vi "svl_Running Equivalent Continuous Sound Level (1 Ch).vi"(6 "integration time [s]":dbl=1.0 format="%.2f", 8 "error in (no error)":errorcluster, 9 "processing state":T1(ring)=enum."Restart averaging", 11 "scaled signal":waveform(dbl)={"t0"=timestamp(0 s since 1904-01-01), "dt"=0.0, "Y"=[]}) -> (0 "error out":errorcluster, 3 "Running Leq":dbl format="%.2f", 4 "actual integration time [s]":dbl=1.0 format="%.2f")   [LabVIEW 2017]
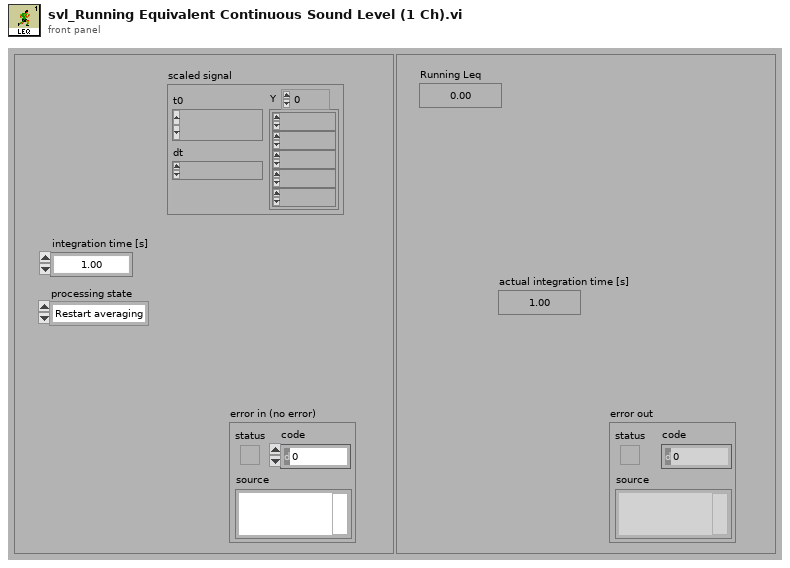
[diagram p1: front panel]
types:
  T1 = enum16{"Reset filter", "Restart averaging", "Continue processing"}
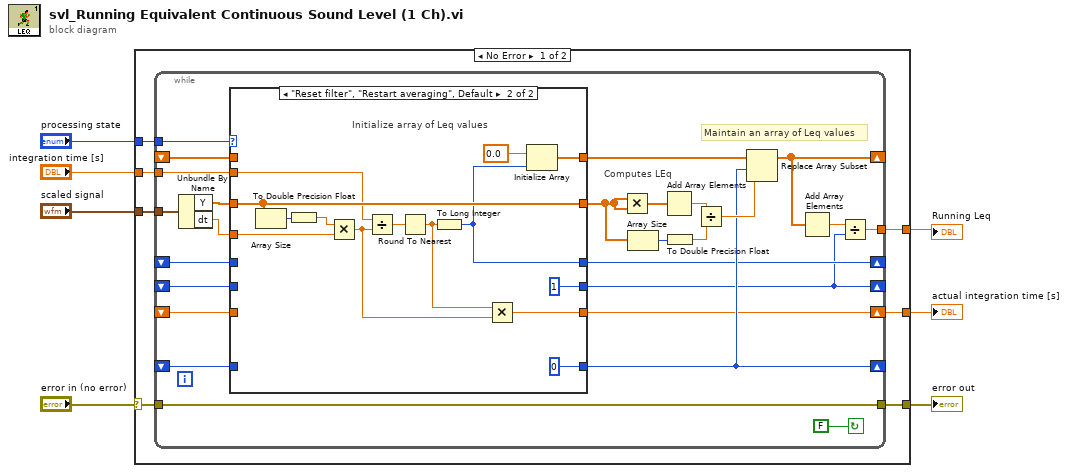
[diagram p0: block diagram]
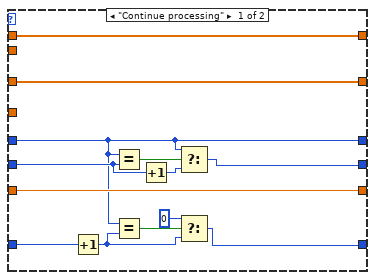
[diagram p2: hidden frame]
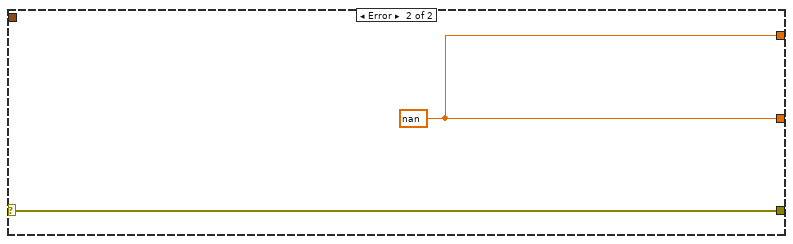
[diagram p3: hidden frame]
diagram:
  n1 = case shown="No Error" "error in (no error)" {
    selector: "error in (no error)" -> [w13 w69]
    tunnel: "integration time [s]" -> [w11 _]
    tunnel: "processing state" -> [w14 _]
    tunnel: [w10 w69] -> w4
    tunnel: [w12 w68] -> w3
    tunnel: [w9 w68] -> w2
    tunnel: "scaled signal" -> [w8 _]
    frame No Error {
      n2 = while {
        shift-left: _ -> [w19]
        shift-right: [w18] -> _
        shift-left: _ -> [w22]
        shift-right: [w23] -> w9
        tunnel: [w21] -> w10
        shift-left: _ -> [w24]
        shift-right: [w20] -> _
        tunnel: w11 -> [w33]
        tunnel: [w39] -> w12
        shift-left: _ -> [w28]
        shift-right: [w25] -> _
        tunnel: w13 -> [w21]
        shift-left: _ -> [w29]
        shift-right: [w26] -> _
        tunnel: w14 -> [w34]
        tunnel: w8 -> [w17]
        stop <- FALSE continue-if-true
        # "Maintain an array of Leq values"
        # "Computes LEq"
        n3 = Unbundle By Name(w17) -> ("Y"=w16:dbl[], "dt"=w15:dbl)
        n4 = case shown="\"Reset filter\", \"Restart averaging\", Default" w34 {
          tunnel: w33 -> [_ w62]
          tunnel: [w52 w65] -> w31
          tunnel: w16 -> [w53 w64]
          tunnel: [w53 w64] -> w30
          tunnel: w15 -> [_ w60]
          tunnel: w29 -> [w52 _]
          tunnel: [w41 0 ("duration (sec)")] -> w25
          tunnel: w28 -> [w48 _]
          tunnel: [w43 1 ("duration (sec)")] -> w18
          tunnel: w24 -> [w42 _]
          tunnel: [w50 w63] -> w23
          tunnel: w22 -> [w50 _]
          tunnel: [w42 w58] -> w20
          tunnel: w19 -> [w44 _]
          frame "Continue processing" {
            n5 = Increment(x=w48) -> (x+1=w47:i32)
            n6 = Equal?(x=w42, y=w44) -> (x = y?=w46:bool)
            n7 = Equal?(x=w42, y=w47) -> (x = y?=w49:bool)
            n8 = Increment(x=w44) -> (x+1=w45:i32)
            n9 = Select(t=w42, s=w46, f=w45) -> (s? t:f=w43:i32)
            n10 = Select(t=0, s=w49, f=w47) -> (s? t:f=w41:i32)
          }
          frame "Reset filter", "Restart averaging", Default {
            # "Initialize array of Leq values"
            n11 = Array Size(array=w64) -> (size(s)=w67:i32)
            n12 = To Double Precision Float(number=w67) -> (double precision float=w55:dbl)
            n13 = Multiply(x=w55, y=w60) -> (x*y=w59:dbl)
            n14 = Divide(x=w62, y=w59) -> (x/y=w61:dbl)
            n15 = Round To Nearest(number=w61) -> (nearest integer value=w54:dbl)
            n16 = To Long Integer(number=w54) -> (32bit integer=w58:i32)
            n17 = Multiply(x=w54, y=w59) -> (x*y=w63:dbl)
            n18 = Initialize Array(0.0 ("duration (sec)"), w58) -> (w65:dbl[])
          }
        }
        n19 = Multiply(x=w30, y=w30) -> (x*y=w32:dbl[])
        n20 = Array Size(array=w30) -> (size(s)=w37:i32)
        n21 = Add Array Elements(numeric array=w32) -> (sum=w38:dbl)
        n22 = To Double Precision Float(number=w37) -> (double precision float=w36:dbl)
        n23 = Divide(x=w38, y=w36) -> (x/y=w35:dbl)
        n24 = Replace Array Subset(array=w31, new element=w35, index=w25) -> (w26:dbl[])
        n25 = Add Array Elements(numeric array=w26) -> (sum=w27:dbl)
        n26 = Divide(x=w27, y=w18) -> (x/y=w39:dbl)
      }
    }
    frame Error {
      w68 = nan
    }
  }
  "error out" <- w4
  "actual integration time [s]" <- w2
  "Running Leq" <- w3
